vi "extract receive info.vi"(1 "Receive data":string) -> (12 "Address":string, 13 "Function Code":string, 14 "STATUS":string, 15 "Feed rate":string)   [LabVIEW 2014, in "HPCNC.lvlib"]
uses:
  HPCNC.lvlib
  GetCncPosition.dll
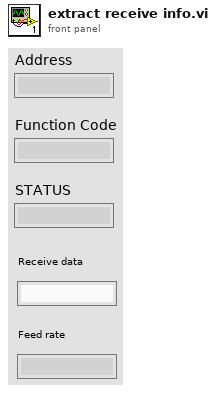
[diagram p1: front panel]
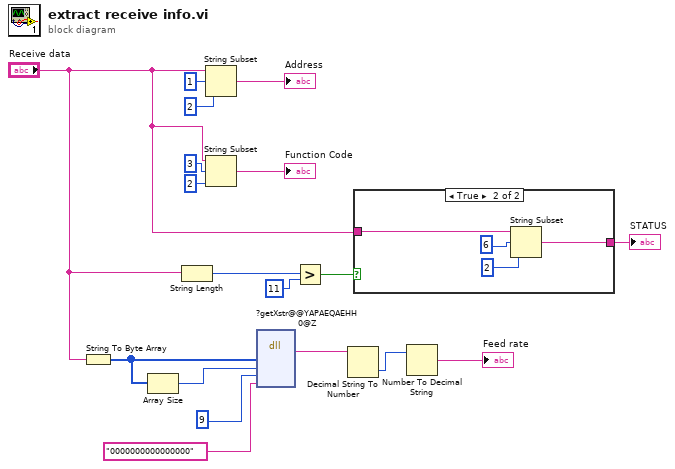
[diagram p0: block diagram]
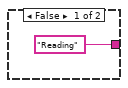
[diagram p2: hidden frame]
diagram:
  n1 = String To Byte Array(string="Receive data") -> (unsigned byte array=w11:u8[])
  n2 = Array Size(array=w11) -> (size(s)=w12:i32)
  n3 = String Length(string="Receive data") -> (length=w5:i32)
  n4 = String Subset(string="Receive data", offset (0)=1, length (rest)=2 ("length (rest)")) -> (substring=→"Address":string)
  n5 = String Subset(string="Receive data", offset (0)=3, length (rest)=2 ("length (rest)")) -> (substring=→"Function Code":string)
  n6 = dll-call lib="D:/Workspace/Giang/Labview/Minigantry With FS/SubVIs/GetCncPosition.dll" fn="?getXstr@@YAPAEQAEHH0@Z" label="Data index"("arrayI"=w11, "size"=w12, "dataToGet"=9, "returnArray"="0000000000000000") -> ("return type"=w8:string)  [unwired: 7 in, 2 out]
  n7 = Greater?(x=w5, y=11) -> (0:w3:bool)
  n8 = Decimal String To Number(string=w8) -> (number=w7:i32)  [unwired: 2 in, 1 out]
  n9 = case shown="True" w3 {
    tunnel: "Receive data" -> [_ w21]
    tunnel: ["Reading" ("StringIn") w20] -> w1
    frame False {
    }
    frame True {
      n10 = String Subset(string=w21, offset (0)=6, length (rest)=2 ("length (rest)")) -> (substring=w20:string)
    }
  }
  "STATUS" <- w1
  n11 = Number To Decimal String(number=w7) -> (decimal integer string=→"Feed rate":string)  [unwired: 1 in]
